vi "ArrangePointsXY.vi"(8 "error in (no error)":errorcluster, 10 "DutyCluster":T1 {"Iteration" items=["first iteration", "second iteration"]}, 11 "XYZ Point coordinates (pixels)":dbl[][](array[numeric])) -> (0 "error out":errorcluster, 2 "DutyCluster":T1 {"Iteration" items=["first iteration", "second iteration"]}, 3 "XYZ Point coordinates updated (pixels)":dbl[][](array[numeric]))   [LabVIEW 2010]
uses:
  TypeDefs/DutyCluster.ctl
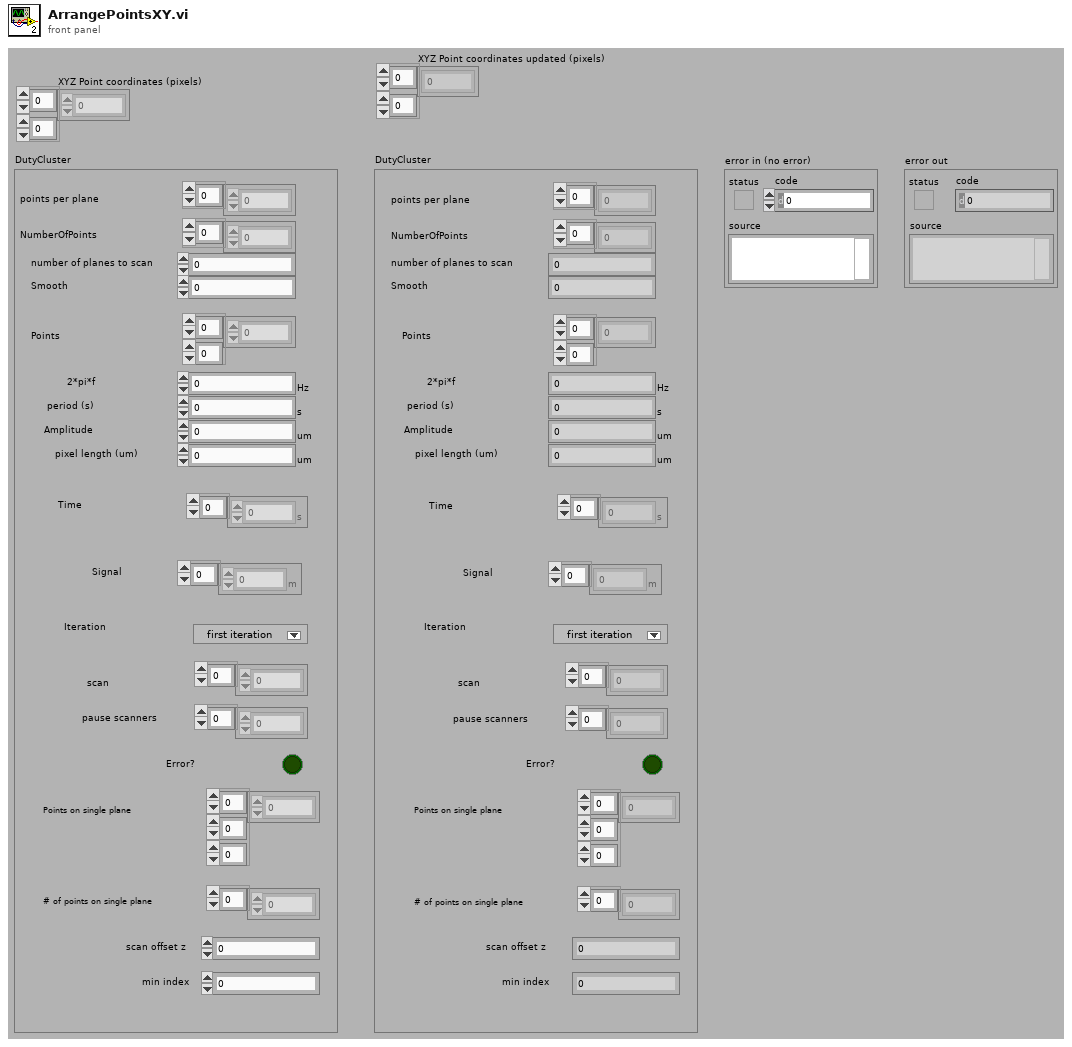
[diagram p1: front panel]
types:
  T1 = typedef "DutyCluster.ctl" = cluster{"points per plane":i32[], "NumberOfPoints":i32[], "number of planes to scan":i32, "Smooth":i32, "Points":dbl[][], "2*pi*f":dbl[unit], "period (s)":dbl[unit], "Amplitude":dbl[unit], "pixel length (um)":dbl[unit], "Time":dbl[unit][], "Signal":dbl[unit][], "Iteration":u16, "scan":i32[], "pause scanners":i32[], "Error?":bool, "Points on single plane":dbl[][][], "# of points on single plane":i32[], "scan offset z":i32, "min index":i32}
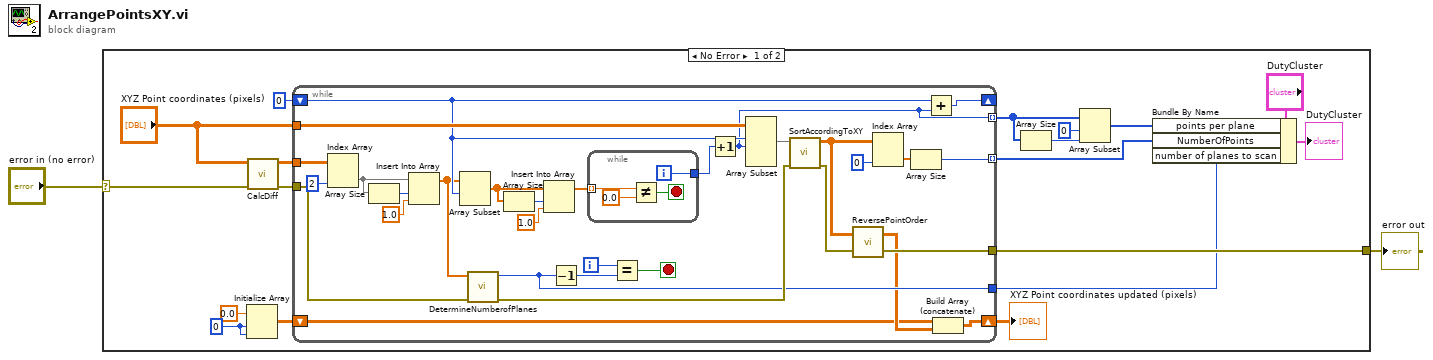
[diagram p0: block diagram]
diagram:
  n1 = case shown="No Error" "error in (no error)" {
    selector: "error in (no error)" -> [w14 w56]
    tunnel: [w13 w56] -> w1
    frame No Error {
      w4 = 0 ("dimension size")
      n2 = Initialize Array(0.0 ("element"), w4, w4) -> (w6:dbl[][])
      n3 = call "CalcDiff.vi"("error in (no error)"=w14, "XYZ Point coordinates (pixels)"="XYZ Point coordinates (pixels)") -> ("error out"=w15:errorcluster, "XYZ Point coordinates (pixels) difference"=w16:dbl[][])  [unwired: 8 in]
      n4 = while {
        tunnel: w16 -> [w50]
        tunnel: "XYZ Point coordinates (pixels)" -> [w49]
        shift-right: [w47] -> _
        shift-left: 0 ("index") -> [w42]
        tunnel: [w24] -> w11 mode=indexing
        tunnel: [w35] -> w19 mode=indexing
        tunnel: w15 -> [w32]
        tunnel: [w29] -> w13
        tunnel: [w26] -> w9
        shift-right: [w22] -> w3
        shift-left: w6 -> [w21]
        i -> [w33]
        stop <- w46 stop-if-true
        n5 = Index Array(array=w50, index (col)=2 ("disabled index (col)")) -> (element=w44:dbl[])  [unwired: 1 in]
        n6 = Array Size(array=w44) -> (size(s)=w45:i32)
        n7 = Insert Into Array(array=w44, index=w45, new element=1.0 ("new element/subarray")) -> (w34:dbl[])
        n8 = Array Subset(array=w34, index=w42) -> (w39:dbl[])  [unwired: 1 in]
        n9 = call "DetermineNumberofPlanes.vi"("error in (no error)"=w32, "Z coordinates (pixels)"=w34) -> ("error out"=w31:errorcluster, "number of planes to scan"=w26:i32)  [unwired: 8 in]
        n10 = Array Size(array=w39) -> (size(s)=w40:i32)
        n11 = Insert Into Array(array=w39, index=w40, new element=1.0 ("new element/subarray")) -> (w38:dbl[])
        n12 = Decrement(x=w26) -> (x-1=w25:i32)
        n13 = while {
          tunnel: w38 -> [w55] mode=indexing
          tunnel: [w52] -> w48
          i -> [w52]
          stop <- w53 stop-if-true
          n14 = Not Equal?(x=w55, y=0.0) -> (x != y?=w53:bool)
        }
        n15 = Equal?(x=w33, y=w25) -> (x = y?=w46:bool)
        n16 = Increment(x=w48) -> (x+1=w35:i32)
        n17 = Array Subset(array=w49, index (row)=w42, length (row)=w35) -> (w27:dbl[][])  [unwired: 2 in]
        n18 = call "SortAccordingToXY.vi"("error in (no error)"=w31, "XYZ Point coordinates (pixels)"=w27) -> ("error out"=w30:errorcluster, "XYZ Point coordinates updated (pixels)"=w28:dbl[][])  [unwired: 8 in]
        n19 = call "ReversePointOrder.vi"("error in (no error)"=w30, "Points In (pixels)"=w28) -> ("error out"=w29:errorcluster, "Points Out (pixels) reversed"=w23:dbl[][])
        n20 = Index Array(array=w28, index (col)=0 ("disabled index (col)")) -> (element=w37:dbl[])  [unwired: 1 in]
        n21 = Array Size(array=w37) -> (size(s)=w24:i32)
        n22 = Add(x=w42, y=w35) -> (x+y=w47:i32)
        n23 = Build Array (concatenate)(w21, w23) -> (w22:dbl[][])
      }
      "XYZ Point coordinates updated (pixels)" <- w3
      n24 = Array Size(array=w19) -> (size(s)=w7:i32)
      n25 = Array Subset(array=w19, index=0, length=w7) -> (w12:i32[])
      n26 = Bundle By Name(cluster="DutyCluster", "points per plane"=w12, "NumberOfPoints"=w11, "number of planes to scan"=w9) -> (→"DutyCluster":T1)
    }
    frame Error {
    }
  }
  "error out" <- w1
